vi "CheckFoderExists.vi"(8 "error in (no error)":errorcluster, 10 "shotnumber":i32, 11 "Input Stripped Path":path) -> (0 "error out":errorcluster)   [LabVIEW 2020, in "BaseDriver.lvclass"]
uses:
  BaseDriver.lvclass
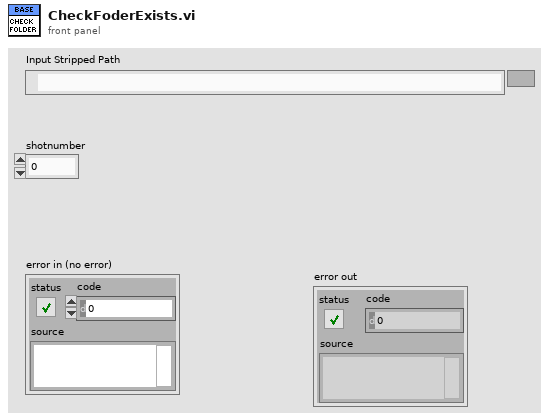
[diagram p1: front panel]
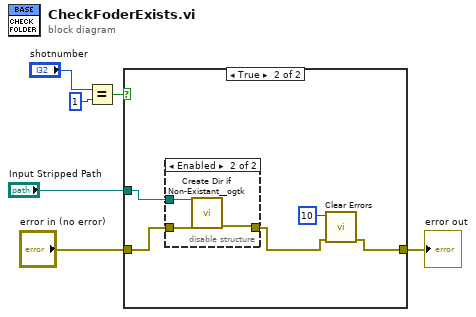
[diagram p0: block diagram]
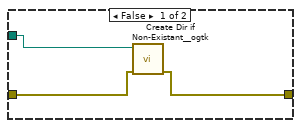
[diagram p2: hidden frame]
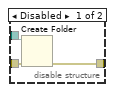
[diagram p3: hidden frame]
diagram:
  n1 = Equal?(x="shotnumber", y=1) -> (x = y?=w4:bool)
  n2 = case shown="True" w4 {
    tunnel: "Input Stripped Path" -> [w9 w14]
    tunnel: "error in (no error)" -> [w8 w13]
    tunnel: [w7 w11] -> w1
    frame False {
      n3 = call <userlib>:"Create Dir if Non-Existant__ogtk.vi"("error in (no error)"=w8, "Directory Path"=w9) -> ("error out"=w7:errorcluster)  [unwired: 7 in, 2 out]
    }
    frame True {
      n4 = disable-structure shown="Enabled" {
        disable-tunnel: w14 -> [w17 w18]
        disable-tunnel: w13 -> [w16 w20]
        disable-tunnel: [w15 w19] -> w12
        frame Disabled {
          n5 = Create Folder(path (use dialog)=w17, error in=w16) -> (error out=w15:errorcluster)  [unwired: 3 out]
        }
        frame Enabled {
          n6 = call <userlib>:"Create Dir if Non-Existant__ogtk.vi"("error in (no error)"=w20, "Directory Path"=w18) -> ("error out"=w19:errorcluster)  [unwired: 7 in, 2 out]
        }
      }
      n7 = call <vilib>:"Clear Errors.vi"("error in (no error)"=w12, "specific error code to clear (0: all)"=10) -> ("error out"=w11:errorcluster)  [unwired: 4 in, 1 out]
    }
  }
  "error out" <- w1
